vi "build token URI.vi"(8 "error in (no error)":errorcluster, 11 "Oauth2.Salesforce in":refnum<class "Oauth2.Salesforce.lvclass">) -> (0 "error out":errorcluster, 1 "Headers":cluster{"header":string, "value":string}[](array[cluster]), 2 "Token Request URI":string, 3 "Oauth2.Salesforce":refnum<class "Oauth2.Salesforce.lvclass">)   [LabVIEW 2017, in "Oauth2.Salesforce.lvclass"]
uses:
  Oauth2.Salesforce.lvclass
  D:/GitHub/Oauth2/source/Oauth2/Oauth2.lvclass
  Oauth2/getTokenElement.vi
  Oauth2/Oauth2.lvclass
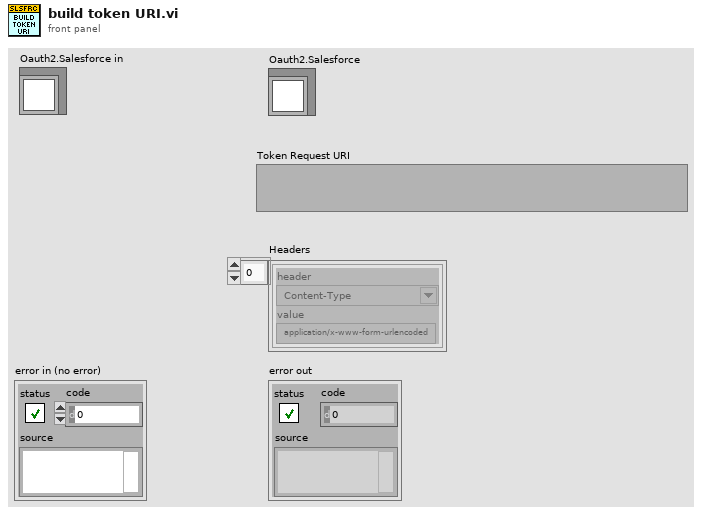
[diagram p1: front panel]
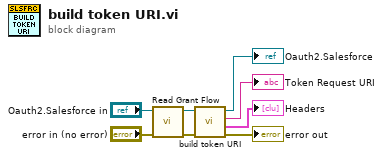
[diagram p0: block diagram]
diagram:
  n1 = call "Read Grant Flow.vi"("error in (no error)"="error in (no error)", "Oauth2 in"="Oauth2.Salesforce in") -> ("error out"=w1:errorcluster, "Oauth2 out"=w3:refnum<class "Oauth2.Salesforce.lvclass">)  [unwired: 7 in, 1 out]
  n2 = call-parent "build token URI.vi"("error in (no error)"=w1, "Oauth2 in"=w3) -> ("error out"=→"error out":errorcluster, "Headers"=→"Headers":cluster{"header":string, "value":string}[], "Token Request URI"=→"Token Request URI":string, "Oauth2"=→"Oauth2.Salesforce":refnum<class "Oauth2.Salesforce.lvclass">)  [unwired: 6 in]
